vi "Get Result.vi"(6 "Last request":bool, 8 "error in (no error)":errorcluster, 11 "Process Object in":refnum<class "Process Object.lvclass">) -> (0 "error out":errorcluster, 2 "Result":refnum<class "Acquired Result.lvclass">, 3 "Process Object out":refnum<class "Process Object.lvclass">)   [LabVIEW 2016, in "Process Object.lvclass"]
uses:
  Process Object.lvclass
  NHMFL_Core/Libraries/Instruments/Results/Acquired Result/Acquired Result.lvclass
  Process Object.lvclass/Process Object.ctl
  Read Result.vi
  Read Result ready.vi
  Worker/Worker.lvclass
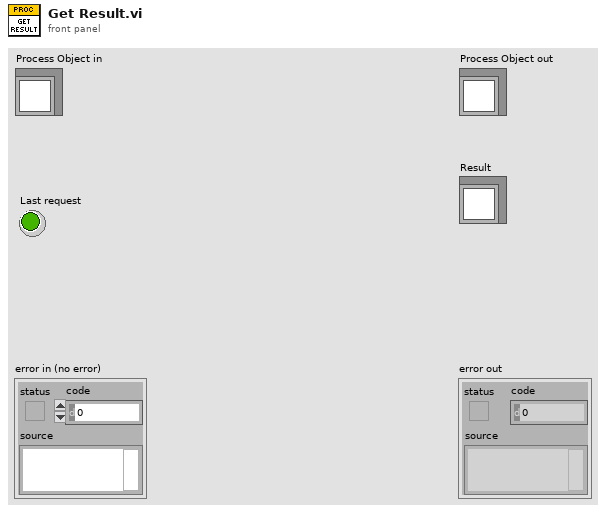
[diagram p1: front panel]
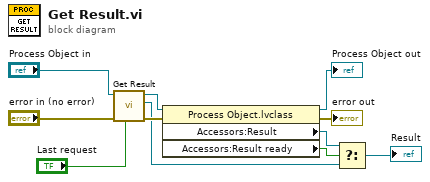
[diagram p0: block diagram]
diagram:
  n1 = call-parent "Get Result.vi"("Last request"="Last request", "error in (no error)"="error in (no error)", "Worker in"="Process Object in") -> ("error out"=w11:errorcluster, "Result"=w1:refnum<class "Acquired Result.lvclass">, "Worker out"=w6:refnum<class "Process Object.lvclass">)  [unwired: 6 in]
  n2 = property class="Process Object.lvclass"(reference=w6, error in=w11) -> (reference out=→"Process Object out":refnum<class "Process Object.lvclass">, error out=→"error out":errorcluster, "Accessors:Result"=w4:refnum<class "Acquired Result.lvclass">, "Accessors:Result ready"=w3:bool)
  n3 = Select(t=w4, s=w3, f=w1) -> (s? t:f=→"Result":refnum<class "Acquired Result.lvclass">)
